vi "metadata_Create.vi"(0 "reference in":refnum<class "metadata.lvclass">, 2 "object name":string, 3 "Metadata":T1, 5 "error in (no error)":errorcluster, 8 "create method":T2=enum."Create or look up existing") -> (14 "reference out":refnum<class "metadata.lvclass">, 19 "error out":errorcluster)   [LabVIEW 2019, in "metadata.lvclass"]
doc: "Constructor."
uses:
  metadata.lvclass
  C:/Program Files/National Instruments/LabVIEW 2019/vi.lib/addons/_AddQ/G#Object/G#Object.lvclass
  <vilib>/addons/_AddQ/G#Object/utils/G#Object_CreateMethod.ctl
  Metadata output --cluster.ctl
  Cantilever info parameters.ctl
  <vilib>/addons/_AddQ/G#Object/G#Object.lvclass
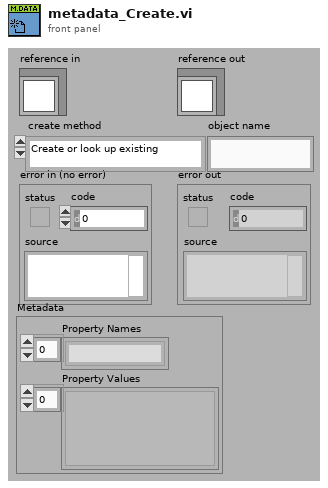
[diagram p1: front panel]
types:
  T1 = typedef "metadata.lvclass/Metadata output --cluster.ctl" = cluster{"Property Names":string[], "Property Values":variant[]}
  T2 = typedef "G#Object.lvclass/G#Object_CreateMethod.ctl" = enum16{"Create", "Create or look up existing", "Look up existing"}
  T3 = typedef "metadata.lvclass/Cantilever info parameters.ctl" = cluster{"spring constant calib method":string, "invOLS calib method":string, "thermal calib deflection channel":string, "model":string, "shape":string, "tip geometry":string, "Laser sum (V)":dbl, "Laser power (mA)":dbl, "invOLS_(nm/V)":dbl, "spring constant nominal (N/m)":dbl, "spring constant calib (N/m)":dbl, "resosnance frequency air calib (Hz)":dbl, "resosnance frequency calib (Hz)":dbl, "quality factor":dbl, "Acoefficident_GCI_(nN.s^1.3/m)":dbl, "half angle (deg)":dbl, "tip radius (m)":dbl, "tip height (m)":dbl, "system mount angle (deg)":dbl}
  T4 = typedef "metadata.lvclass/ObjectAttributesRef.ctl" = refnum<data-value>
  T5 = typedef "metadata.lvclass/ObjectAttributes.ctl" = cluster{"MyAttribute":dbl, "System Control":T6, "file info":T7, "Sample info":T8, "Cantilever info":T3, "XYZ piezos":T9, "Mapping":T10, "Fcurve segment":T11[], "Fast fpga segment":T13, "Chirp":T14, "precision (6)":i16, "width (-)":i16, "Metadata":T1, "config filepath":path, "Section names []":string[], "Property names []":string[], "nb elements":u16}
  T6 = typedef "metadata.lvclass/System control parameters.ctl" = cluster{"FPGA SW version":string, "TDMS file version":string, "Instrument":string, "Instrument model":string, "Instrument scanner":string, "Instrument clockrate (Mhz)":string, "Instrument tick time (us)":string}
  T7 = typedef "metadata.lvclass/File info parameters.ctl" = cluster{"Time Stamp":timestamp, "Filename":string, "Filepath":path, "User":string, "Experiment_name":string, "Curve_id":string, "number_segments":u8, "number_consecutive_scans":u32}
  T8 = typedef "metadata.lvclass/Sample info parameters.ctl" = cluster{"Sample name":string, "Sample species":string}
  T9 = typedef "metadata.lvclass/XYZ piezos parameters.ctl" = cluster{"X stage piezo sensitivity (nm/V)":dbl, "X stage piezo gain":dbl, "X velocity (V/tick)":dbl, "X closed loop":bool, "Y stage piezo sensitivity (nm/V)":dbl, "Y stage piezo gain":dbl, "Y velocity (V/tick)":dbl, "Y closed loop":bool, "Z stage piezo sensitivity (nm/V)":dbl, "Z stage piezo gain":dbl, "Z closed loop":bool, "X position (V)":dbl, "Y position (V)":dbl}
  T10 = typedef "metadata.lvclass/Mapping parameters.ctl" = cluster{"Mapping":bool, "index":u16, "position row":u16, "position column":u16, "next position row":i16, "next position column":i16, "X initial position (V)":dbl, "Y initial position (V)":dbl, "X step size (V)":dbl, "Y step size (V)":dbl}
  T11 = typedef "metadata.lvclass/Fcurve segment.ctl" = cluster{"type":T12, "fast_fpga_trigger":bool, "nb":u8, "duration (ticks)":i64, "nb points":i32, "sampling rate (S/s)":u32, "Zpiezo control out":string, "initial deflection (V)":dbl, "relative setpoint":bool, "setpoint on":bool, "setpoint (V)":dbl, "setpoint trigger channel":string, "velocity (V/tick)":dbl, "Z position setpoint trigger (V)":dbl, "Z retract length (V)":dbl, "dec factor":u32}
  T12 = typedef "metadata.lvclass/Segment type--combobox.ctl" = string
  T13 = typedef "metadata.lvclass/fast fpga segment parameters.ctl" = cluster{"Fast start time trigger":timestamp, "nb_points":u32, "sampling_rate_(S/s)":u32, "duration_(ticks)":u32}
  T14 = typedef "metadata.lvclass/Chirp added parameters.ctl" = cluster{"f start (Hz)":dbl, "f end (Hz)":dbl, "Sweep type":string}
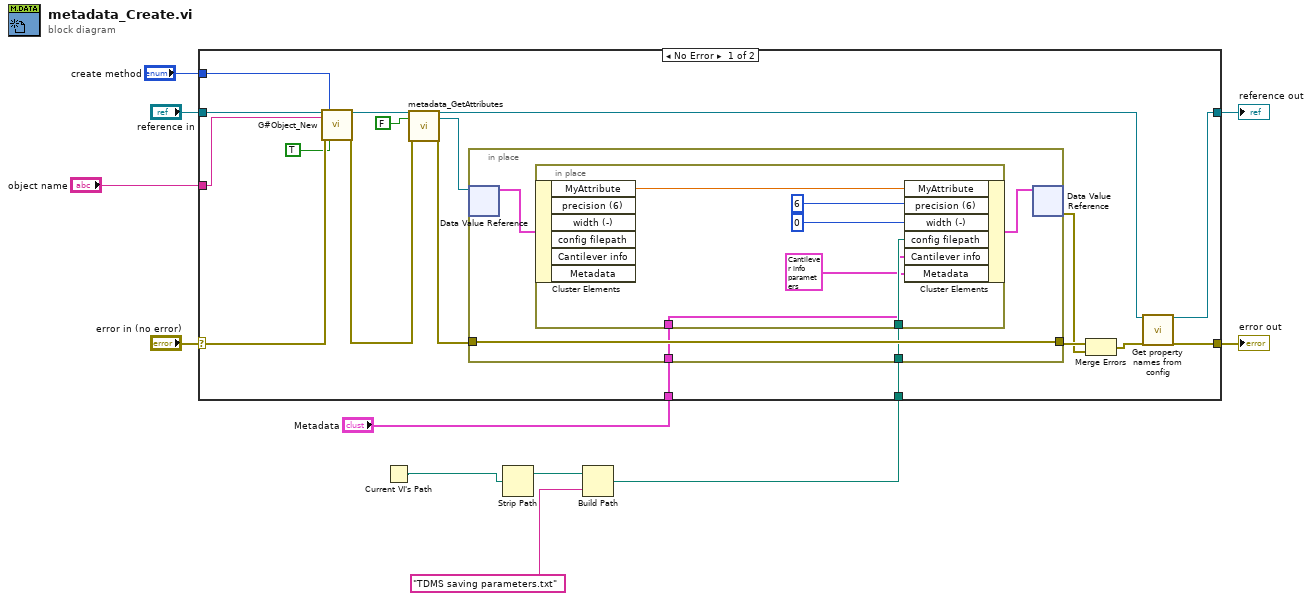
[diagram p0: block diagram]
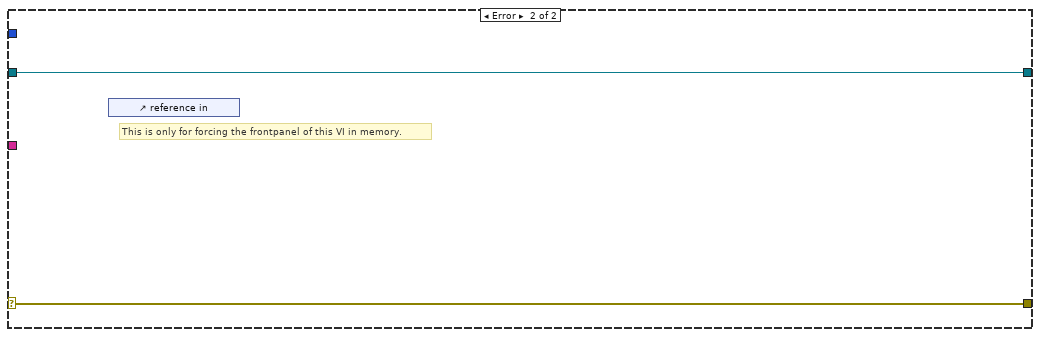
[diagram p2: hidden frame]
diagram:
  n1 = Current VI's Path() -> (path=w4:path)
  n2 = Strip Path(path=w4) -> (stripped path=w7:path)  [unwired: 1 out]
  n3 = Build Path(base path=w7, name or relative path="TDMS saving parameters.txt") -> (appended path=w5:path)
  n4 = case shown="No Error" "error in (no error)" {
    selector: "error in (no error)" -> [w28 w42]
    tunnel: [w15 w42] -> w10
    tunnel: [w13 w41] -> w8
    tunnel: "reference in" -> [w29 w41]
    tunnel: w5 -> [w19 _]
    tunnel: "create method" -> [w18 _]
    tunnel: "object name" -> [w17 _]
    tunnel: "Metadata" -> [w12 _]
    frame No Error {
      n5 = call <vilib>:"G#Object_New.vi"("reference in"=w29, "object name"=w17, "error in (no error)"=w28, "create method"=w18, "user counter (T)?"=TRUE ("User Counter")) -> ("reference out"=w24:refnum<class "metadata.lvclass">, "error out"=w23:errorcluster)  [unwired: 12 in, 1 out]
      n6 = call "metadata_GetAttributes.vi"("reference in"=w24, "return data? (T)"=FALSE ("return data"), "error in (no error)"=w23) -> ("reference out"=w14:refnum<class "metadata.lvclass">, "attributes ref"=w21:T4, "error out"=w22:errorcluster)  [unwired: 13 in, 1 out]
      n7 = in-place {
        in-place-border: w22 -> [w32]
        in-place-border: [w32] -> w26
        in-place-border: w19 -> [w31]
        in-place-border: w12 -> [w30]
        n8 = in-place-dvr #1(w21) -> (w33:T5)  [unwired: 1 out]
        n9 = in-place {
          in-place-border: w31 -> [w37]
          in-place-border: w30 -> [w35]
          n10 = in-place-cluster #2(w33) -> ("MyAttribute"=w40:dbl)  [unwired: 5 out]
          n11 = in-place-cluster #2("MyAttribute"=w40, "precision (6)"=i16 6, "width (-)"=i16 0, "config filepath"=w37, "Cantilever info"=T3 {"spring constant calib method"="Thermal-Sader", "invOLS calib method"="Thermal-Sader", "thermal calib deflection channel"="Deflection_quotient_(V)", "model"="", "shape"="", "tip geometry"="", "Laser sum (V)"=0.0, "Laser power (mA)"=0.0, "invOLS_(nm/V)"=0.0, "spring constant nominal (N/m)"=0.0, "spring constant calib (N/m)"=0.0, "resosnance frequency air calib (Hz)"=0.0, "resosnance frequency calib (Hz)"=0.0, "quality factor"=0.0, "Acoefficident_GCI_(nN.s^1.3/m)"=0.0, "half angle (deg)"=0.0, "tip radius (m)"=0.0, "tip height (m)"=0.0, "system mount angle (deg)"=0.0}, "Metadata"=w35) -> (w34:T5)
        }
        n12 = in-place-dvr #1(w34) -> (w25:errorcluster)  [unwired: 1 out]
      }
      n13 = Merge Errors(w26, w25) -> (w16:errorcluster)
      n14 = call-dynamic "Get property names from config.vi"("reference in"=w14, "error in (no error)"=w16) -> ("reference out"=w13:refnum<class "metadata.lvclass">, "error out"=w15:errorcluster)  [unwired: 13 in, 3 out]
    }
    frame Error {
      # "This is only for forcing the frontpanel of this VI in memory."
      n15 = control-ref of="reference in"() -> ()  [unwired: 1 out]
    }
  }
  "error out" <- w10
  "reference out" <- w8
